vi "SDO_TRAJECTORY_EXECUTE_REL.vi"(6 "EnableClosedLoop":bool=TRUE, 8 "Init":bool, 10 "End Relative\nOrientation Deg":dbl, 11 "Gyro Heading\nRAD":dbl) -> (0 "AtReference":bool, 3 "Chassis Velocity Target":T1 {"vOmega" format="%10.3f"; "vY" format="%10.3f"; "vX" format="%10.3f"})   [LabVIEW 2019]
uses:
  <vilib>/Rock Robotics/WPI/ThirdParty/JAS_Junk/TrajLib/TypeDef/CHASSIS_SPEEDS.ctl
  <vilib>/Rock Robotics/WPI/ThirdParty/JAS_Junk/TrajLib/VI/Util_GetTime_U32.vi
  <vilib>/Rock Robotics/WPI/ThirdParty/JAS_Junk/TrajLib/ProfiledPIDController_NewPeriod.vi
  <vilib>/Rock Robotics/WPI/ThirdParty/JAS_Junk/TrajLib/ProfiledPIDController_SetIntegratorRange.vi
  <vilib>/Rock Robotics/WPI/ThirdParty/JAS_Junk/TrajLib/ProfiledPIDController_DisableContInput.vi
  <vilib>/Rock Robotics/WPI/ThirdParty/JAS_Junk/TrajLib/ProfiledPIDController_EnableContInput.vi
  <vilib>/Rock Robotics/WPI/ThirdParty/JAS_Junk/TrajLib/TrapProfConstraint_New.vi
  <vilib>/Rock Robotics/WPI/ThirdParty/JAS_Junk/TrajLib/SwerveOdometry_UpdateX.vi
  <vilib>/Rock Robotics/WPI/ThirdParty/JAS_Junk/TrajLib/SwerveOdometry_ResetPosition.vi
  <vilib>/Rock Robotics/WPI/ThirdParty/JAS_Junk/TrajLib/SwerveOdometry_New.vi
  <vilib>/Rock Robotics/WPI/ThirdParty/JAS_Junk/TrajLib/HolDrvCtrl_New.vi
  <vilib>/Rock Robotics/WPI/ThirdParty/JAS_Junk/TrajLib/HolDrvCtrl_PackPID.vi
  <vilib>/Rock Robotics/WPI/ThirdParty/JAS_Junk/TrajLib/HolDrvCtrl_SetTolerance.vi
  <vilib>/Rock Robotics/WPI/ThirdParty/JAS_Junk/TrajLib/HolDrvCtrl_SetEnabled.vi
  <vilib>/Rock Robotics/WPI/ThirdParty/JAS_Junk/TrajLib/HolDrvCtrl_Calculate_Trajectory.vi
  <vilib>/Rock Robotics/WPI/ThirdParty/JAS_Junk/TrajLib/HolDrvCtrl_AtReference.vi
  <vilib>/Rock Robotics/WPI/ThirdParty/JAS_Junk/TrajLib/TrapProfState_New.vi
  <vilib>/Rock Robotics/WPI/ThirdParty/JAS_Junk/TrajLib/PIDController_NewPeriod.vi
  <vilib>/Rock Robotics/SystemInterfaces/NetworkCommunication/NetComm_UsageReport_report.vi
  <vilib>/Rock Robotics/WPI/ThirdParty/JAS_Junk/TrajLib/PIDController_SetIntegratorRange.vi
  <vilib>/Rock Robotics/WPI/ThirdParty/JAS_Junk/TrajLib/PIDController_DisableContinousInput.vi
  <vilib>/Rock Robotics/WPI/ThirdParty/JAS_Junk/TrajLib/PIDController_EnableContinousInput.vi
  <vilib>/Rock Robotics/WPI/ThirdParty/JAS_Junk/TrajLib/Rotation2d_Plus.vi
  <vilib>/Rock Robotics/WPI/ThirdParty/JAS_Junk/TrajLib/Twist2d_Create.vi
  <vilib>/Rock Robotics/WPI/ThirdParty/JAS_Junk/TrajLib/Rotation2d_Minus.vi
  <vilib>/Rock Robotics/WPI/ThirdParty/JAS_Junk/TrajLib/Pose2d_getTranslation.vi
  <vilib>/Rock Robotics/WPI/ThirdParty/JAS_Junk/TrajLib/Pose2d_New_TRRO.vi
  <vilib>/Rock Robotics/WPI/ThirdParty/JAS_Junk/TrajLib/VI/SwerveModulePosition_Get.vi
  <vilib>/Rock Robotics/WPI/ThirdParty/JAS_Junk/TrajLib/VI/SwerveModulePosition_New.vi
  <vilib>/Rock Robotics/WPI/ThirdParty/JAS_Junk/TrajLib/Twist2d_GetAll.vi
  <vilib>/Rock Robotics/WPI/ThirdParty/JAS_Junk/TrajLib/Pose2d_getRotation.vi
  <vilib>/Rock Robotics/WPI/ThirdParty/JAS_Junk/TrajLib/Conv_Deg_Radians.vi
  <vilib>/Rock Robotics/WPI/ThirdParty/JAS_Junk/TrajLib/PIDController_Reset.vi
  <vilib>/Rock Robotics/WPI/ThirdParty/JAS_Junk/TrajLib/HolDrvCtrl_Calculate.vi
  <vilib>/Rock Robotics/WPI/ThirdParty/JAS_Junk/TrajLib/Pose2d_getXYAngle.vi
  <vilib>/Rock Robotics/WPI/ThirdParty/JAS_Junk/TrajLib/Rotation2d_GetRadians.vi
  <vilib>/Rock Robotics/WPI/ThirdParty/JAS_Junk/TrajLib/Rotation2d_RotateBy.vi
  <vilib>/Rock Robotics/WPI/ThirdParty/JAS_Junk/TrajLib/Rotation2d_UnaryMinus.vi
  <vilib>/Rock Robotics/WPI/ThirdParty/JAS_Junk/TrajLib/Rotation2d_GetAngleCosSin.vi
  <vilib>/Rock Robotics/WPI/ThirdParty/JAS_Junk/TrajLib/Pose2d_RelativeTo.vi
  <vilib>/Rock Robotics/WPI/ThirdParty/JAS_Junk/TrajLib/ProfiledPIDController_Calculate_Meas_Goal.vi
  <vilib>/Rock Robotics/WPI/ThirdParty/JAS_Junk/TrajLib/ChassisSpeeds_FromFieldRelativeSpeeds.vi
  <vilib>/Rock Robotics/WPI/ThirdParty/JAS_Junk/TrajLib/PIDController_Calculate_SP_PV.vi
  <vilib>/Rock Robotics/WPI/ThirdParty/JAS_Junk/TrajLib/ProfiledPIDController_Reset_PosOnly.vi
  <vilib>/Rock Robotics/WPI/ThirdParty/JAS_Junk/TrajLib/Rotation2d_CreateXY.vi
  <vilib>/Rock Robotics/WPI/ThirdParty/JAS_Junk/TrajLib/Transform2d_Create_PosePose.vi
  <vilib>/Rock Robotics/WPI/ThirdParty/JAS_Junk/TrajLib/ProfiledPIDController_SetGoal_PosOnly.vi
  <vilib>/Rock Robotics/WPI/ThirdParty/JAS_Junk/TrajLib/ProfiledPIDController_Calculate_Meas.vi
  <vilib>/Rock Robotics/WPI/ThirdParty/JAS_Junk/TrajLib/Rotation2d_GetCos.vi
  <vilib>/Rock Robotics/WPI/ThirdParty/JAS_Junk/TrajLib/Rotation2d_GetSin.vi
  <vilib>/Rock Robotics/WPI/ThirdParty/JAS_Junk/TrajLib/PIDController_SetSetpoint.vi
  <vilib>/Rock Robotics/WPI/ThirdParty/JAS_Junk/TrajLib/PIDController_Calculate_PV.vi
  <vilib>/Rock Robotics/WPI/ThirdParty/JAS_Junk/TrajLib/ProfiledPIDController_Reset.vi
  <vilib>/Rock Robotics/WPI/ThirdParty/JAS_Junk/TrajLib/Util_CalcDist.vi
  <vilib>/Rock Robotics/WPI/ThirdParty/JAS_Junk/TrajLib/Translation2d_RotateBy.vi
  <vilib>/Rock Robotics/WPI/ThirdParty/JAS_Junk/TrajLib/Translation2d_Minus.vi
  <vilib>/Rock Robotics/WPI/ThirdParty/JAS_Junk/TrajLib/ProfiledPIDController_SetGoal.vi
  <vilib>/Rock Robotics/WPI/ThirdParty/JAS_Junk/TrajLib/TrapProfile_New.vi
  <vilib>/Rock Robotics/WPI/ThirdParty/JAS_Junk/TrajLib/ProfiledPIDController_GetPeriod.vi
  <vilib>/Rock Robotics/WPI/ThirdParty/JAS_Junk/TrajLib/TrapProfile_Calculate.vi
  <vilib>/Rock Robotics/WPI/ThirdParty/JAS_Junk/TrajLib/ControllerUtil_GetModulusError.vi
  <vilib>/Rock Robotics/WPI/ThirdParty/JAS_Junk/TrajLib/Translation2d_Create.vi
  <vilib>/Rock Robotics/WPI/ThirdParty/JAS_Junk/TrajLib/TrapProfile_ShouldFlipAcceleration.vi
  <vilib>/Rock Robotics/WPI/ThirdParty/JAS_Junk/TrajLib/TrapProfile_Direct.vi
  <vilib>/Rock Robotics/WPI/ThirdParty/JAS_Junk/TrajLib/PIDController_GetPeriod.vi
  Swerve_Drive_System/SDO_DRIVE_GLOBALS.vi
  <vilib>/Rock Robotics/WPI/ThirdParty/JAS_Junk/TrajLib/VI/Util_GetTime_U64.vi
  SDO_TRAJECTORY_GLOBALS.vi
  <vilib>/Rock Robotics/WPI/ThirdParty/JAS_Junk/TrajLib/Globals/Util_LibraryGlobals.vi
  <vilib>/Rock Robotics/WPI/ThirdParty/JAS_Junk/TrajLib/VI/SwerveKinematics_ToTwist2dX.vi
  <vilib>/Rock Robotics/WPI/ThirdParty/JAS_Junk/TrajLib/Pose2d_Exp.vi
  <vilib>/Rock Robotics/WPI/ThirdParty/JAS_Junk/TrajLib/Trajectory_Library.lvlib
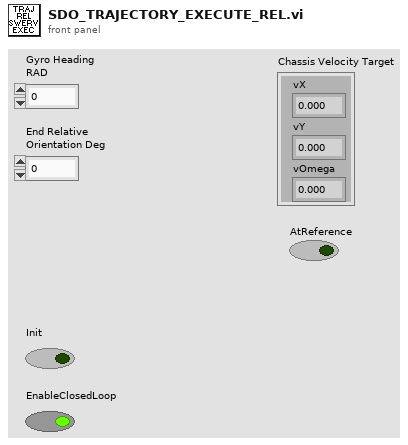
[diagram p1: front panel]
types:
  T1 = typedef "Trajectory_Library.lvlib/CHASSIS_SPEEDS.ctl" = cluster{"vX":dbl, "vY":dbl, "vOmega":dbl}
  T2 = typedef "Trajectory_Library.lvlib/ROTATION2D.ctl" = cluster{"VALUE":dbl, "COS":dbl, "SIN":dbl}
  T3 = typedef "Trajectory_Library.lvlib/SWERVE_DRIVE_KINEMATICS.ctl" = cluster{"NumModules":i32, "InverseKinematics":T4, "ForwardKinematics":T4, "Modules":T5[], "PrevCoR":T5, "SavedModuleStates":T6[]}
  T4 = typedef "NI_Matrix.lvlib/RealMatrix.ctl" = dbl[][]
  T5 = typedef "Trajectory_Library.lvlib/TRANSLATION2D.ctl" = cluster{"X":dbl, "Y":dbl}
  T6 = typedef "Trajectory_Library.lvlib/SWERVE_DRIVE_MODULE_STATE.ctl" = cluster{"Speed":dbl, "Angle":T2}
  T7 = typedef "Trajectory_Library.lvlib/SWERVE_DRIVE_MODULE_POSITION.ctl" = cluster{"Distance":dbl, "Angle":T2, "P":bool}
  T8 = typedef "Trajectory_Library.lvlib/TRAJECTORY.ctl" = cluster{"TotalTImeSecs":dbl, "States":T9[]}
  T9 = typedef "Trajectory_Library.lvlib/TRAJ_STATE.ctl" = cluster{"TimeSeconds":dbl, "Velocity":dbl, "Acceleration":dbl, "POSE":T10, "Curvature":dbl}
  T10 = typedef "Trajectory_Library.lvlib/POSE2D.ctl" = cluster{"TRANSLATION":T5, "ROTATION":T2}
  T11 = typedef "Trajectory_Library.lvlib/PID_TUNING.ctl" = cluster{"Kp":dbl, "Ki":dbl, "Kd":dbl, "MaximumIntegral":dbl, "MinimumIntegral":dbl}
  T12 = typedef "Trajectory_Library.lvlib/PROFILED_PID_CONTROLLER.ctl" = cluster{"Controller":T13, "Goal":T14, "Setpoint":T14, "Constraint":T15}
  T13 = typedef "Trajectory_Library.lvlib/PID_CONTROLLER.ctl" = cluster{"Kp":dbl, "Ki":dbl, "Kd":dbl, "Period":dbl, "Max_Integral":dbl, "Min_Integral":dbl, "Max_Input":dbl, "Min_Input":dbl, "Continuous":bool, "PositionError":dbl, "VelocityError":dbl, "PrevError":dbl, "TotalError":dbl, "PositionTolerance":dbl, "VelocityTolerance":dbl, "SetPoint":dbl, "Kf":dbl, "Prev_Deriv":dbl, "Prev_Deriv 2":dbl, "DerivativeFilter":bool, "Min_Output":dbl, "Max_Output":dbl, "Prev_F_P":dbl, "Prev_F_P_2":dbl, "AntiWindupActive":bool, "Measurement":dbl}
  T14 = typedef "Trajectory_Library.lvlib/TRAPEZOID_PROFILE_STATE.ctl" = cluster{"Position":dbl, "Velocity":dbl}
  T15 = typedef "Trajectory_Library.lvlib/TRAPEZOID_PROFILE_CONSTRAINT.ctl" = cluster{"MaxVelocity":dbl, "MaxAcceleration":dbl}
  T16 = typedef "Trajectory_Library.lvlib/HOLONOMIC_PACK_TUNING.ctl" = cluster{"X PID Tuning":T11, "Y PID Tuning":T11, "thetaProfiledPID_CTRL":T12}
  T17 = typedef "Trajectory_Library.lvlib/HOLONOMIC_DRV_CTRL.ctl" = cluster{"poseTolerance":T10, "poseError":T10, "Enabled":bool, "PID_xCtrl":T13, "PID_yCtrl":T13, "PROF_PID_thetaCtrl":T12, "RotationError":T2, "FirstRun":bool}
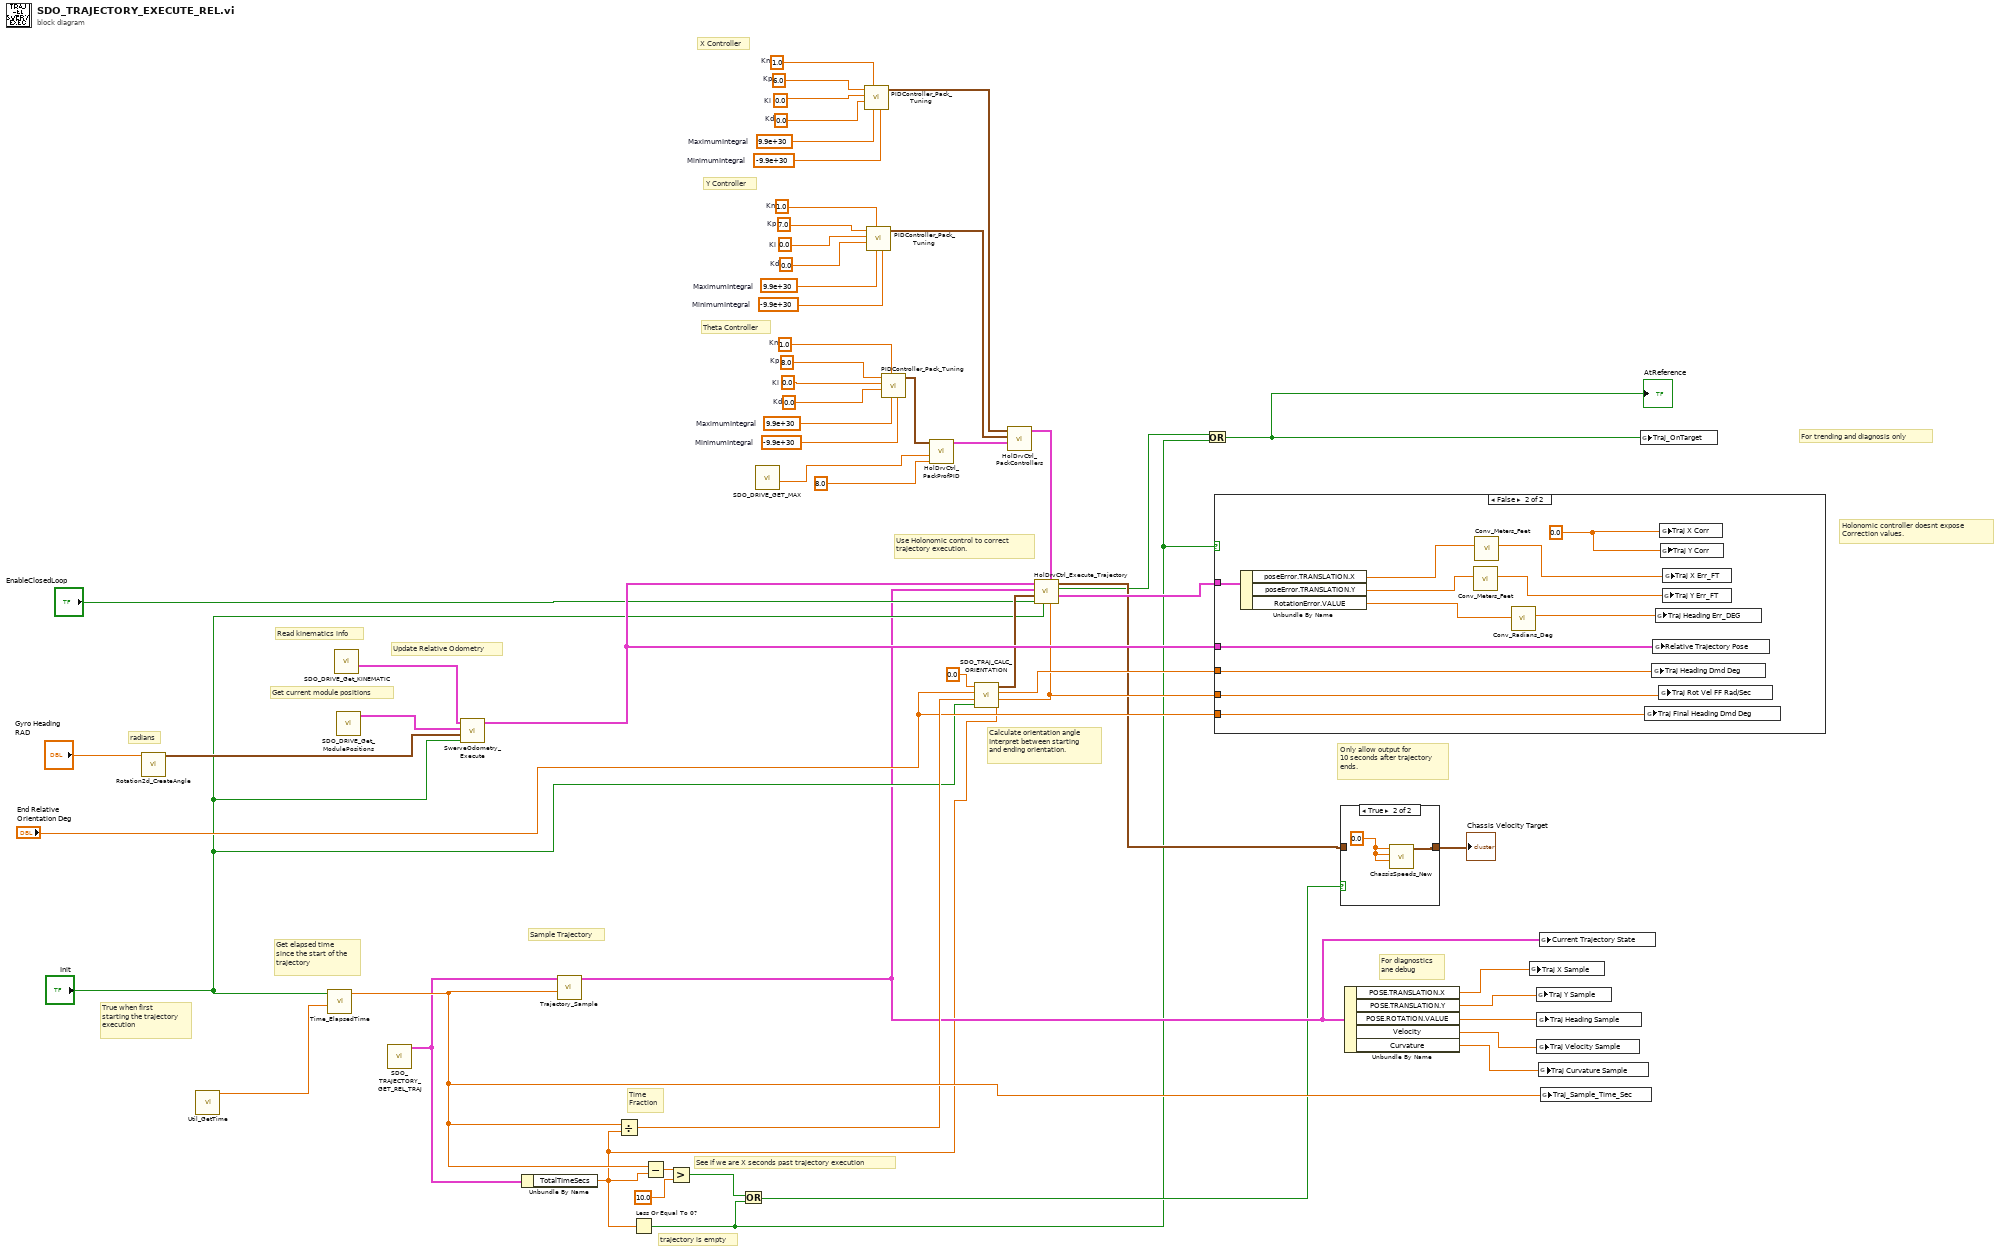
[diagram p0: block diagram]
diagram:
  w23 = 1.0  # Kn
  w26 = 8.0  # Kp
  w35 = 0.0  # Ki
  w36 = 0.0  # Kd
  w37 = 9.9e+30  # MaximumIntegral
  w38 = -9.9e+30  # MinimumIntegral
  w21 = 1.0  # Kn
  w24 = 6.0  # Kp
  w27 = 0.0  # Ki
  w28 = 0.0  # Kd
  w29 = 9.9e+30  # MaximumIntegral
  w30 = -9.9e+30  # MinimumIntegral
  w22 = 1.0  # Kn
  w25 = 7.0  # Kp
  w31 = 0.0  # Ki
  w32 = 0.0  # Kd
  w33 = 9.9e+30  # MaximumIntegral
  w34 = -9.9e+30  # MinimumIntegral
  # "trajectory is empty"
  # "Theta Controller"
  # "Y Controller"
  # "X Controller"
  # "Time\nFraction"
  # "Calculate orientation angle\nInterpret between starting\nand ending orientation."
  # "Get current module positions"
  # "True when first\nstarting the trajectory\nexecution"
  # "Get elapsed time\nsince the start of the\ntrajectory"
  # "Holonomic controller doesnt expose\nCorrection values."
  # "Use Holonomic control to correct\ntrajectory execution."
  # "For trending and diagnosis only"
  # "For diagnostics\nane debug"
  # "Update Relative Odometry"
  # "Read kinematics info"
  # "Sample Trajectory"
  # "See if we are X seconds past trajectory execution"
  # "radians"
  # "Only allow output for\n10 seconds after trajectory\nends."
  n1 = call <vilib>:"Rotation2d_CreateAngle.vi"("Angle"="Gyro Heading\nRAD") -> ("ROTATION"=w54:T2)  [unwired: 10 in]
  n2 = call <vilib>:"Util_GetTime.vi"() -> ("FPGA_Time_Seconds"=w52:dbl)  [unwired: 9 in, 2 out]
  n3 = call <vilib>:"Time_ElapsedTime.vi"("PassthroughTime_SEC"=w52, "Reset"="Init") -> ("Elapsed Time Sec"=w45:dbl)  [unwired: 9 in]
  n4 = call "SDO_DRIVE_Get_KINEMATIC.vi"() -> ("out SWERVE_DRIVE_KINEMATICS"=w8:T3)  [unwired: 11 in]
  n5 = call "SDO_DRIVE_Get_ModulePositions.vi"() -> ("Swerve Module Positions"=w53:T7[])  [unwired: 11 in]
  n6 = call "SDO_TRAJECTORY_GET_REL_TRAJ.vi"() -> ("Relative_Trajectory"=w10:T8)  [unwired: 11 in]
  n7 = call <vilib>:"SwerveOdometry_Execute.vi"("Init"="Init", "Rotation"=w54, "Swerve Module Positions"=w53, "SWERVE_DRIVE_KINEMATICS"=w8) -> ("Current Pose"=w19:T10)  [unwired: 5 in, 2 out]
  n8 = Unbundle By Name(w10) -> ("TotalTImeSecs"=w6:dbl)
  n9 = call <vilib>:"Trajectory_Sample.vi"("Time"=w45, "InputTRAJECTORY"=w10) -> ("OutputTRAJ_STATE"=w9:T9)  [unwired: 9 in]
  n10 = Divide(x=w45, y=w6) -> (x/y=w44:dbl)
  n11 = Less Or Equal To 0?(x=w6) -> (x <= 0?=w1:bool)
  n12 = Subtract(x=w45, y=w6) -> (x-y=w58:dbl)
  n13 = Greater?(x=w58, y=10.0) -> (0:w5:bool)
  n14 = Or(x=w5, y=w1) -> (x .or. y?=w4:bool)
  n15 = call "SDO_DRIVE_GET_MAX.vi"() -> ("Max Rotational Vel (Rad/Sec)"=w12:dbl)  [unwired: 10 in, 1 out]
  n16 = call <vilib>:"PIDController_Pack_Tuning.vi"("MinimumIntegral"=w30, "MaximumIntegral"=w29, "Kn"=w21, "Kd"=w28, "Ki"=w27, "Kp"=w24) -> ("PID Tuning"=w39:T11)  [unwired: 5 in]
  n17 = call <vilib>:"PIDController_Pack_Tuning.vi"("MinimumIntegral"=w34, "MaximumIntegral"=w33, "Kn"=w22, "Kd"=w32, "Ki"=w31, "Kp"=w25) -> ("PID Tuning"=w40:T11)  [unwired: 5 in]
  n18 = call <vilib>:"PIDController_Pack_Tuning.vi"("MinimumIntegral"=w38, "MaximumIntegral"=w37, "Kn"=w23, "Kd"=w36, "Ki"=w35, "Kp"=w26) -> ("PID Tuning"=w20:T11)  [unwired: 5 in]
  n19 = call <vilib>:"HolDrvCtrl_PackProfPID.vi"("Max Accel"=8.0, "Max Speed"=w12, "Theta PID Tuning"=w20) -> ("Theta PID CONTROLLER"=w41:T12)  [unwired: 8 in]
  n20 = call "SDO_TRAJ_CALC_ORIENTATION.vi"("Total Trajectory Time"=w6, "Init"="Init", "Time Fraction"=w44, "End Orientation Demand DEG"="End Relative\nOrientation Deg", "Starting Orientation  DEG"=0.0) -> ("Rotational Velocity Rad Per Sec"=w15:dbl, 2:"Orientation Demand Deg"=w46:dbl, 3:"Orientation Demand Deg"=w18:T2)  [unwired: 4 in]
  n21 = call <vilib>:"HolDrvCtrl_PackControllers.vi"("thetaProfiledPID_CTRL"=w41, "Y PID Tuning"=w40, "X PID Tuning"=w39) -> ("HOLONOMIC_CTRL_PACK_TUNING"=w42:T16)  [unwired: 8 in]
  n22 = call <vilib>:"HolDrvCtrl_Execute_Trajectory.vi"("Rotational Velocity Feedforward \nRad/Sec"=w15, "HOLONOMIC_CTRL_PACK_TUNING"=w42, "Reset"="Init", "Enable"="EnableClosedLoop", "angleRef"=w18, "desiredTrajState"=w9, "currentPose"=w19) -> ("outHOLONOMIC_DRV_CTRL"=w17:T17, "AtReference"=w3:bool, "calcChassisSpeed"=w7:T1)  [unwired: 2 in]
  n23 = Or(x=w3, y=w1) -> (x .or. y?=w2:bool)
  "AtReference" <- w2
  n24 = case shown="False" w1 {
    tunnel: w46 -> [_ w69]
    tunnel: "End Relative\nOrientation Deg" -> [_ w68]
    tunnel: w19 -> [_ w62]
    tunnel: w17 -> [_ w61]
    tunnel: w15 -> [_ w60]
    frame True {
    }
    frame False {
      w70 = 0.0 ("Y Corr")
      n25 = Unbundle By Name(w61) -> ("poseError.TRANSLATION.X"=w66:dbl, "poseError.TRANSLATION.Y"=w65:dbl, "RotationError.VALUE"=w59:dbl)
      n26 = call <vilib>:"Conv_Meters_Feet.vi"("Meters"=w65) -> ("Feet"=w64:dbl)  [unwired: 10 in]
      n27 = call <vilib>:"Conv_Meters_Feet.vi"("Meters"=w66) -> ("Feet"=w63:dbl)  [unwired: 10 in]
      n28 = call <vilib>:"Conv_Radians_Deg.vi"("Radians"=w59) -> ("Degrees"=w67:dbl)  [unwired: 10 in]
      n29 = global write "SDO_TRAJECTORY_GLOBALS.vi" "Traj Final Heading Dmd Deg"(w68) -> ()
      n30 = global write "SDO_TRAJECTORY_GLOBALS.vi" "Traj Heading Dmd Deg"(w69) -> ()
      n31 = global write "SDO_TRAJECTORY_GLOBALS.vi" "Relative Trajectory Pose"(w62) -> ()
      n32 = global write "SDO_TRAJECTORY_GLOBALS.vi" "Traj Heading Err_DEG"(w67) -> ()
      n33 = global write "SDO_TRAJECTORY_GLOBALS.vi" "Traj Rot Vel FF Rad/Sec"(w60) -> ()
      n34 = global write "SDO_TRAJECTORY_GLOBALS.vi" "Traj X Corr"(w70) -> ()
      n35 = global write "SDO_TRAJECTORY_GLOBALS.vi" "Traj Y Corr"(w70) -> ()
      n36 = global write "SDO_TRAJECTORY_GLOBALS.vi" "Traj Y Err_FT"(w64) -> ()
      n37 = global write "SDO_TRAJECTORY_GLOBALS.vi" "Traj X Err_FT"(w63) -> ()
    }
  }
  n38 = case shown="True" w4 {
    tunnel: w7 -> [w71 _]
    tunnel: [w71 w72] -> w55
    frame False {
    }
    frame True {
      w73 = 0.0 ("vX")
      n39 = call <vilib>:"ChassisSpeeds_New.vi"("vAngular"=w73, "vY"=w73, "vX"=w73) -> ("CHASSIS"=w72:T1)  [unwired: 8 in]
    }
  }
  "Chassis Velocity Target" <- w55
  n40 = Unbundle By Name(w9) -> ("POSE.TRANSLATION.X"=w51:dbl, "POSE.TRANSLATION.Y"=w50:dbl, "POSE.ROTATION.VALUE"=w49:dbl, "Velocity"=w48:dbl, "Curvature"=w47:dbl)
  n41 = global write "SDO_TRAJECTORY_GLOBALS.vi" "Traj X Sample"(w51) -> ()
  n42 = global write "SDO_TRAJECTORY_GLOBALS.vi" "Traj Y Sample"(w50) -> ()
  n43 = global write "SDO_TRAJECTORY_GLOBALS.vi" "Traj Heading Sample"(w49) -> ()
  n44 = global write "SDO_TRAJECTORY_GLOBALS.vi" "Traj Velocity Sample"(w48) -> ()
  n45 = global write "SDO_TRAJECTORY_GLOBALS.vi" "Traj Curvature Sample"(w47) -> ()
  n46 = global write "SDO_TRAJECTORY_GLOBALS.vi" "Current Trajectory State"(w9) -> ()
  n47 = global write "SDO_TRAJECTORY_GLOBALS.vi" "Traj_Sample_Time_Sec"(w45) -> ()
  n48 = global write "SDO_TRAJECTORY_GLOBALS.vi" "Traj_OnTarget"(w2) -> ()
